vi "MH_GetDebugInfo.vi"(8 "error in (no error)":errorcluster, 11 "devidx":i32) -> (0 "error out":errorcluster, 2 "debuginfo":string, 3 "return type":i32)   [LabVIEW 2019]
uses:
  MH_DllPath_global.vi
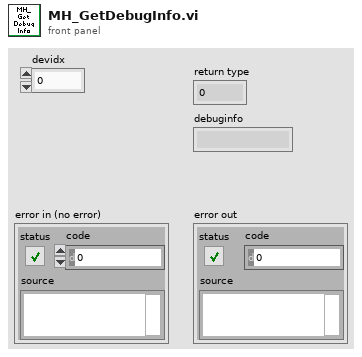
[diagram p1: front panel]
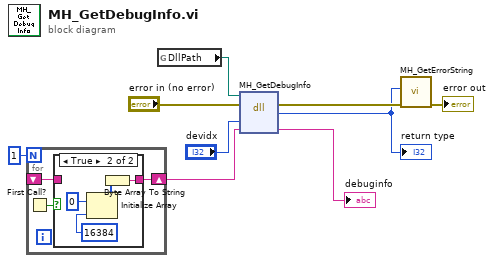
[diagram p0: block diagram]
diagram:
  n1 = for {
    N: 1 -> [_]
    shift-right: [w11] -> w1
    shift-left: _ -> [w10]
    n2 = First Call?() -> (First Call?: T/F=w12:bool)
    n3 = case shown="True" w12 {
      tunnel: [w13 w14] -> w11
      tunnel: w10 -> [w13 _]
      frame False {
      }
      frame True {
        n4 = Initialize Array(u8 0, 16384 ("dimension size")) -> (w15:u8[])
        n5 = Byte Array To String(unsigned byte array=w15) -> (string=w14:string)
      }
    }
  }
  n6 = global read "MH_DllPath_global.vi" "DllPath"() -> (w7:path)
  n7 = dll-call lib="MHLib64.dll" fn="MH_GetDebugInfo"(path in=w7, error in="error in (no error)", "devidx"="devidx", "debuginfo"=w1) -> (error out=w6:errorcluster, "return type"=w5:i32, "debuginfo"=→"debuginfo":string)  [unwired: 2 in, 1 out]
  "return type" <- w5
  n8 = call "MH_GetErrorString.vi"("error in (no error)"=w6, "code"=w5) -> ("error out"=→"error out":errorcluster)  [unwired: 7 in, 2 out]
